vi "Test_move_2D.vi"() -> ()   [LabVIEW 2019]
panel:
  in  "Acceleration":u16
  in  "Address y":u8
  in  "Address x":u8
  in  "Target y":i32
  in  "Speed":i16
  in  "Target x":i32
  in  "COM Port for serial\nconnection. Check device\nmanager.":string
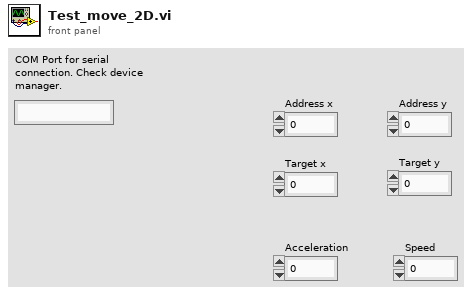
[diagram p1: front panel]
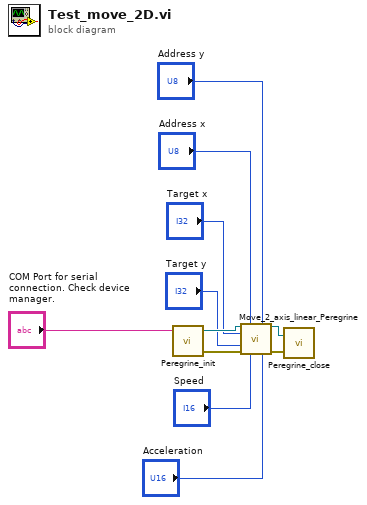
[diagram p0: block diagram]
diagram:
  n1 = call "Peregrine_init.vi"("COM Port for serial\nconnection. Check device\nmanager."="COM Port for serial\nconnection. Check device\nmanager.") -> ("error out"=w9:errorcluster, "Handle out"=w10:refnum<visa-resource-name>)  [unwired: 3 in]
  n2 = call "Move_2_axis_linear_Peregrine.vi"("Handle in"=w10, "Address x"="Address x", "Address y"="Address y", "Target x"="Target x", "Target y"="Target y", "error"=w9, "Speed"="Speed", "Acceleration"="Acceleration") -> ("Handle out"=w8:refnum<visa-resource-name>, "error out"=w7:errorcluster)  [unwired: 6 in]
  n3 = call "Peregrine_close.vi"("error in (no error)"=w7, "Handle in"=w8) -> ()  [unwired: 1 in, 1 out]
